vi "Проверка Витерби 1.vi"() -> ()   [LabVIEW 2012]
uses:
  Global 1.vi
  <vilib>/ptbypt/NI_PtbyPt.lvlib
panel:
  out "x/y":dbl
  in  "Запуск\nкомб ус-ва":bool
  in  "standard deviation":dbl(knob)=0.6170110432045905 scale=0.0..1.0
  in  "stop":bool
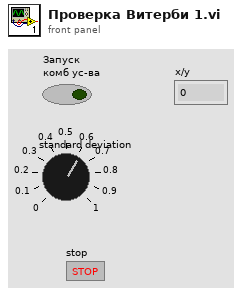
[diagram p1: front panel]
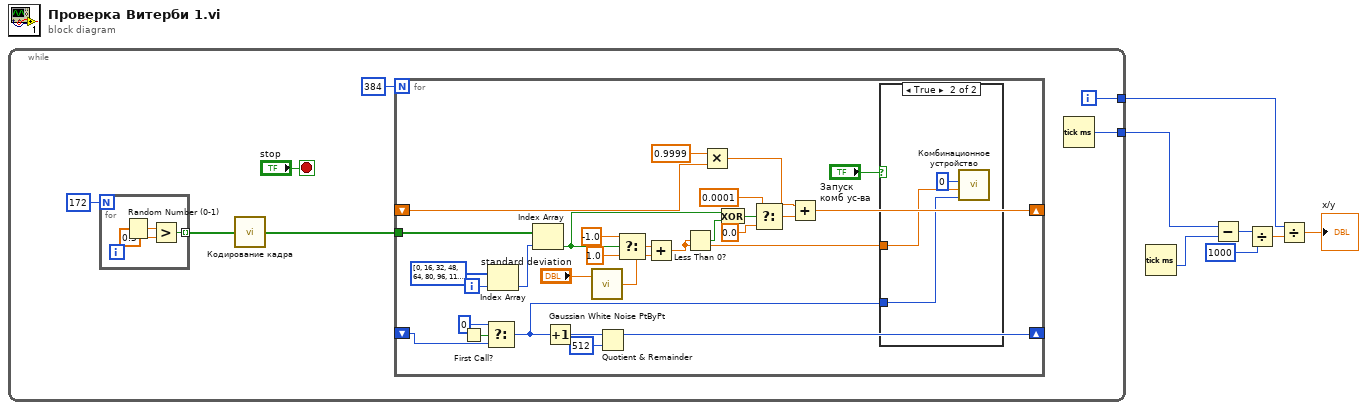
[diagram p0: block diagram]
diagram:
  n1 = while {
    tunnel: [w9] -> w3
    tunnel: [w8] -> w1
    i -> [w8]
    stop <- "stop" stop-if-true
    n2 = for {
      N: 172 -> [_]
      tunnel: [w15] -> w10 mode=indexing
      n3 = Random Number (0-1)() -> (number: 0 to 1=w16:dbl)
      n4 = Greater?(x=w16, y=0.5) -> (0:w15:bool)
    }
    n5 = call "Кодирование кадра.vi"("Кадр на вход\nкодера"=w10) -> ("Поток кодированных \nбитов"=w14:bool[])  [unwired: 14 in]
    n6 = for {
      N: 384 -> [_]
      tunnel: w14 -> [w37]
      shift-right: [w33] -> _
      shift-left: _ -> [w20]
      shift-right: [w23] -> _
      shift-left: _ -> [w22]
      i -> [w40]
      n7 = First Call?() -> (First Call?: T/F=w18:bool)
      n8 = Select(t=0, s=w18, f=w20) -> (s? t:f=w21:i32)
      n9 = Index Array(array=i32[] [0, 16, 32, 48, 64, 80, 96, 112, 128, 144, 160, 176, 192, 208, 224, 240, 256, 272, 288, 304, 320, 336, 352, 368, 1, 17, 33, 49, 65, 81, 97, 113, 129, 145, 161, 177, 193, 209, 225, 241, 257, 273, 289, 305, 321, 337, 353, 369, 2, 18, 34, 50, 66, 82, 98, 114, 130, 146, 162, 178, 194, 210, 226, 242, 258, 274, 290, 306, 322, 338, 354, 370, 3, 19, 35, 51, 67, 83, 99, 115, 131, 147, 163, 179, 195, 211, 227, 243, 259, 275, 291, 307, 323, 339, 355, 371, 4, 20, 36, 52, 68, 84, 100, 116, 132, 148, 164, 180, 196, 212, 228, 244, 260, 276, 292, 308, 324, 340, 356, 372, 5, 21, 37, 53, 69, 85, 101, 117, 133, 149, 165, 181, 197, 213, 229, 245, 261, 277, 293, 309, 325, 341, 357, 373, 6, 22, 38, 54, 70, 86, 102, 118, 134, 150, 166, 182, 198, 214, 230, 246, 262, 278, 294, 310, 326, 342, 358, 374, 7, 23, 39, 55, 71, 87, 103, 119, 135, 151, 167, 183, 199, 215, 231, 247, 263, 279, 295, 311, 327, 343, 359, 375, 8, 24, 40, 56, 72, 88, 104, 120, 136, 152, 168, 184, 200, 216, 232, 248, 264, 280, 296, 312, 328, 344, 360, 376, 9, 25, 41, 57, 73, 89, 105, 121, 137, 153, 169, 185, 201, 217, 233, 249, 265, 281, 297, 313, 329, 345, 361, 377, 10, 26, 42, 58, 74, 90, 106, 122, 138, 154, 170, 186, 202, 218, 234, 250, 266, 282, 298, 314, 330, 346, 362, 378, 11, 27, 43, 59, 75, 91, 107, 123, 139, 155, 171, 187, 203, 219, 235, 251, 267, 283, 299, 315, 331, 347, 363, 379, 12, 28, 44, 60, 76, 92, 108, 124, 140, 156, 172, 188, 204, 220, 236, 252, 268, 284, 300, 316, 332, 348, 364, 380, 13, 29, 45, 61, 77, 93, 109, 125, 141, 157, 173, 189, 205, 221, 237, 253, 269, 285, 301, 317, 333, 349, 365, 381, 14, 30, 46, 62, 78, 94, 110, 126, 142, 158, 174, 190, 206, 222, 238, 254, 270, 286, 302, 318, 334, 350, 366, 382, 15, 31, 47, 63, 79, 95, 111, 127, 143, 159, 175, 191, 207, 223, 239, 255, 271, 287, 303, 319, 335, 351, 367, 383] ("Сформированный массив 2"), index=w40) -> (element=w38:i32)
      n10 = Index Array(array=w37, index=w38) -> (element=w30:bool)
      n11 = Increment(x=w21) -> (x+1=w34:i32)
      n12 = call <vilib>:"Gaussian White Noise PtByPt.vi"("standard deviation"="standard deviation") -> ("Gaussian white noise"=w42:dbl)  [unwired: 2 in]
      n13 = Quotient & Remainder(x=w34, y=512) -> (x-y*floor(x/y)=w33:i32)  [unwired: 1 out]
      n14 = Select(t=-1.0, s=w30, f=1.0) -> (s? t:f=w45:dbl)
      n15 = Add(x=w45, y=w42) -> (x+y=w31:dbl)
      n16 = Less Than 0?(x=w31) -> (x < 0?=w32:bool)
      n17 = Multiply(x=0.9999, y=w22) -> (x*y=w25:dbl)
      n18 = Exclusive Or(1:w32, 2:w30) -> (0:w29:bool)
      n19 = Select(t=0.0001, s=w29, f=0.0) -> (s? t:f=w26:dbl)
      n20 = Add(x=w25, y=w26) -> (x+y=w23:dbl)
      n21 = case shown="True" "Запуск\nкомб ус-ва" {
        tunnel: w31 -> [_ w47]
        tunnel: w21 -> [_ w46]
        frame False {
        }
        frame True {
          n22 = call "Комбинационное устройство.vi"("НОМЕР БИТА"=w46, "Значение пика"=w47, "НОМЕР ЛУЧА"=0) -> ()  [unwired: 9 in]
        }
      }
    }
    n23 = Tick Count (ms)() -> (millisecond timer value=w9:u32)
  }
  n24 = Tick Count (ms)() -> (millisecond timer value=w2:u32)
  n25 = Subtract(x=w3, y=w2) -> (x-y=w7:u32)
  n26 = Divide(x=w7, y=u32 1000) -> (x/y=w5:dbl)
  n27 = Divide(x=w1, y=w5) -> (x/y=→"x/y":dbl)
